vi "InvFilter-Create Noise.vi"(0 "Calibration File":path, 1 "seed":i32=37, 5 "Noise In":dbl[](array[numeric]), 7 "InvFilt Params":T2={"Min Frequency (Hz)"=0.0, "Max Frequency (Hz)"=0.0, "Length (points)"=301, "Sampling rate (Hz)"=0.0, "Delay (ms)"=301.0, "Linear phase"=FALSE}, 9 "Brickwall (T)":bool=TRUE, 11 "error in (no error)":errorcluster) -> (3 "Mag Spec":T1, 4 "InvFilter Noise":dbl[](array[numeric]), 8 "Max Level":dbl, 15 "error out":errorcluster)   [LabVIEW 2020]
uses:
  InvFilt-Params.ctl
  epl-vi-lib/PXI DAQ VIs/DAQ Engine VIs/PXI Globals.vi
  epl-vi-lib/Signal Synthesis VIs/Waveform VIs/Noise VIs/Noise-Globals.vi
  epl-vi-lib/Utility VIs/Math VIs/FFT x(t) to dB,Degrees (1D).vi
  epl-vi-lib/Utility VIs/Math VIs/Linear to dB (scalar).vi
  <vilib>/Analysis/NI_AALBase.lvlib
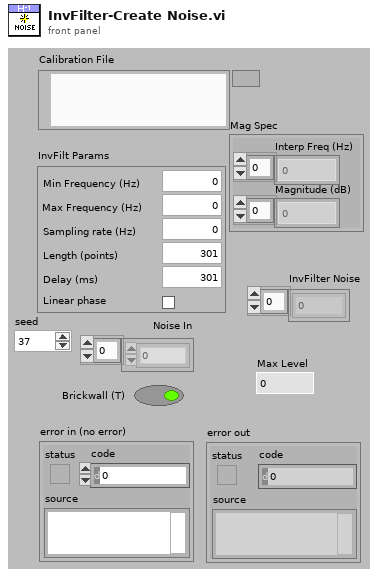
[diagram p1: front panel]
types:
  T1 = cluster{"Interp Freq (Hz)":dbl[], "Magnitude (dB)":dbl[]}
  T2 = typedef "InvFilt-Params.ctl" = cluster{"Min Frequency (Hz)":dbl, "Max Frequency (Hz)":dbl, "Length (points)":i32, "Sampling rate (Hz)":dbl, "Delay (ms)":dbl, "Linear phase":bool}
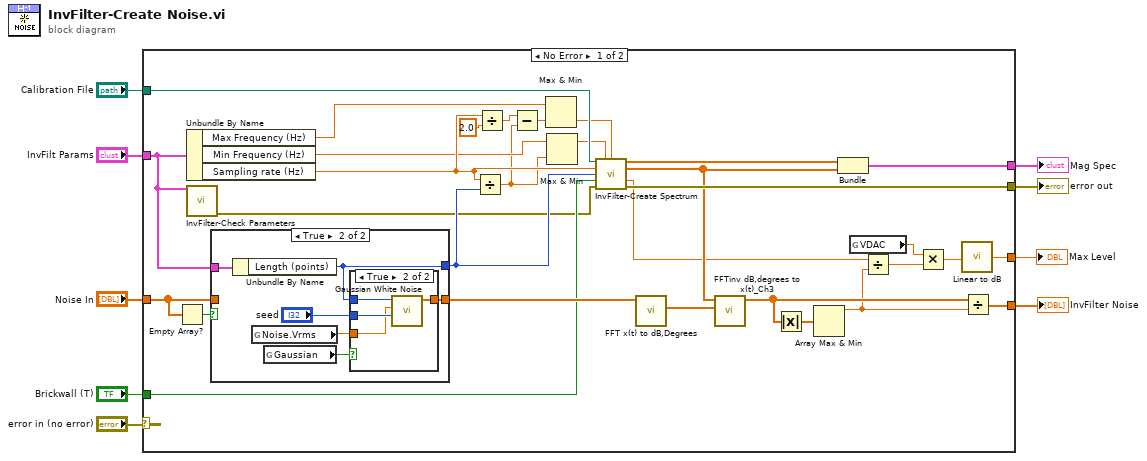
[diagram p0: block diagram]
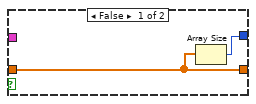
[diagram p2: hidden frame]
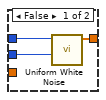
[diagram p3: hidden frame]
diagram:
  n1 = case shown="No Error" "error in (no error)" {
    selector: "error in (no error)" -> [_ w56]
    tunnel: [w39 w56] -> w8
    tunnel: "Calibration File" -> [w40 _]
    tunnel: "InvFilt Params" -> [w11 _]
    tunnel: [w37 _] -> w5
    tunnel: [w38 _] -> w4
    tunnel: "Noise In" -> [w21 _]
    tunnel: "Brickwall (T)" -> [w20 _]
    tunnel: [w18 _] -> w1
    frame No Error {
      n2 = Empty Array?(array=w21) -> (empty?=w24:bool)
      n3 = Unbundle By Name(w11) -> ("Max Frequency (Hz)"=w36:dbl, "Min Frequency (Hz)"=w32:dbl, "Sampling rate (Hz)"=w33:dbl)
      n4 = call "InvFilter-Check Parameters.vi"("InvFilt Params"=w11) -> ("error out"=w10:errorcluster)  [unwired: 14 in]
      n5 = case shown="True" w24 {
        tunnel: w11 -> [_ w48]
        tunnel: [w42 w46] -> w23
        tunnel: [w41 w47] -> w22
        tunnel: w21 -> [w41 _]
        frame False {
          n6 = Array Size(array=w41) -> (size(s)=w42:i32)
        }
        frame True {
          n7 = Unbundle By Name(w48) -> ("Length (points)"=w46:i32)
          n8 = global read "Noise-Globals.vi" "Noise.Vrms"() -> (w43:dbl)
          n9 = global read "Noise-Globals.vi" "Gaussian"() -> (w44:bool)
          n10 = case shown="True" w44 {
            tunnel: [w51 w55] -> w47
            tunnel: w46 -> [w50 w54]
            tunnel: "seed" -> [w49 w53]
            tunnel: w43 -> [_ w52]
            frame False {
              n11 = call <vilib>:"Uniform White Noise.vi"("seed"=w49, "samples"=w50) -> ("uniform white noise"=w51:dbl[])  [unwired: 8 in, 1 out]
            }
            frame True {
              n12 = call <vilib>:"Gaussian White Noise.vi"("seed"=w53, "standard deviation"=w52, "samples"=w54) -> ("Gaussian noise pattern"=w55:dbl[])  [unwired: 7 in, 1 out]
            }
          }
        }
      }
      n13 = Divide(x=w33, y=w23) -> (x/y=w31:dbl)
      n14 = Divide(x=w33, y=2.0) -> (x/y=w29:dbl)
      n15 = Subtract(x=w29, y=w31) -> (x-y=w34:dbl)
      n16 = Max & Min(x=w36, y=w34) -> (min(x,y)=w35:dbl)  [unwired: 1 out]
      n17 = Max & Min(x=w32, y=w31) -> (max(x,y)=w30:dbl)  [unwired: 1 out]
      n18 = call "InvFilter-Create Spectrum.vi"("Calibration file"=w40, "Fmin (Hz)"=w30, "Fmax (Hz)"=w35, "Fs (Hz)"=w33, "Npts"=w23, "Brickwall (T)"=w20, "error in (no error)"=w10) -> ("Interp Freq (Hz)"=w14:dbl[], "Magnitude (dB)"=w13:dbl[], "reference"=w12:dbl, "error out"=w39:errorcluster)  [unwired: 4 in, 1 out]
      n19 = call-poly "FFT x(t) to dB,Degrees.vi"("X"=w22) -> ("+Freq Phase of FFT (degrees)"=w27:dbl[])  [unwired: 8 in, 2 out]
      n20 = call "FFTinv dB,degrees to x(t)_Ch3.vi"("+Freq Phase of FFT (degrees)"=w27, "+Freq. Mag of FFT (rms dB)"=w13) -> ("X(t)"=w25:dbl[])  [unwired: 8 in, 1 out]
      n21 = Absolute Value(x=w25) -> (abs(x)=w26:dbl[])
      n22 = Array Max & Min(array=w26) -> (max value=w17:dbl)  [unwired: 3 out]
      n23 = Bundle("Interp Freq (Hz)"=w14, "Magnitude (dB)"=w13) -> (w38:T1)  [unwired: 1 in]
      n24 = global read "PXI Globals.vi" "VDAC"() -> (w15:dbl)
      n25 = Divide(x=w12, y=w17) -> (x/y=w19:dbl)
      n26 = Multiply(x=w15, y=w19) -> (x*y=w16:dbl)
      n27 = call-poly "Linear to dB.vi"("Linear"=w16) -> ("dB"=w18:dbl)
      n28 = Divide(x=w25, y=w17) -> (x/y=w37:dbl[])
    }
    frame Error {
    }
  }
  "error out" <- w8
  "InvFilter Noise" <- w5
  "Mag Spec" <- w4
  "Max Level" <- w1
